vi "DPO 4034 Config Channel.vi"(4 "Bandwidth (0: FULL)":u16(ring) items=["FULL", "250 MHz", "150 MHz", "20 MHz"], 5 "Input Impedance (0: 1M ohm)":u16(ring) items=["1M", "75", "50"], 6 "Vertical Range (10.0 V)":dbl=10.0, 7 "Enable Channel (T: Enable)":bool=TRUE, 8 "error in (no error)":errorcluster, 9 "Vertical Coupling (1: DC)":u16(ring)=1 items=["AC", "DC", "Ground"], 10 "Channel (0: Channel 1)":u16(ring) items=["Channel 1", "Channel 2", "Channel 3", "Channel 4", "Math", "Reference 1", "Reference 2", "Reference 3", "Reference 4", "Bus 1", "Bus 2"], 11 "VISA resource name":refnum<visa-resource-name>) -> (0 "error out":errorcluster, 3 "VISA resource name out":refnum<visa-resource-name>)   [LabVIEW 2012]
panel:
  in  "Vertical Offset (0.0 V)":dbl
  in  "Probe Attenuation (1)":dbl=1.0
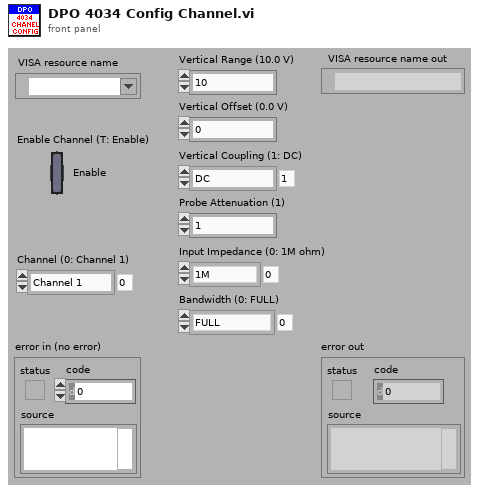
[diagram p1: front panel]
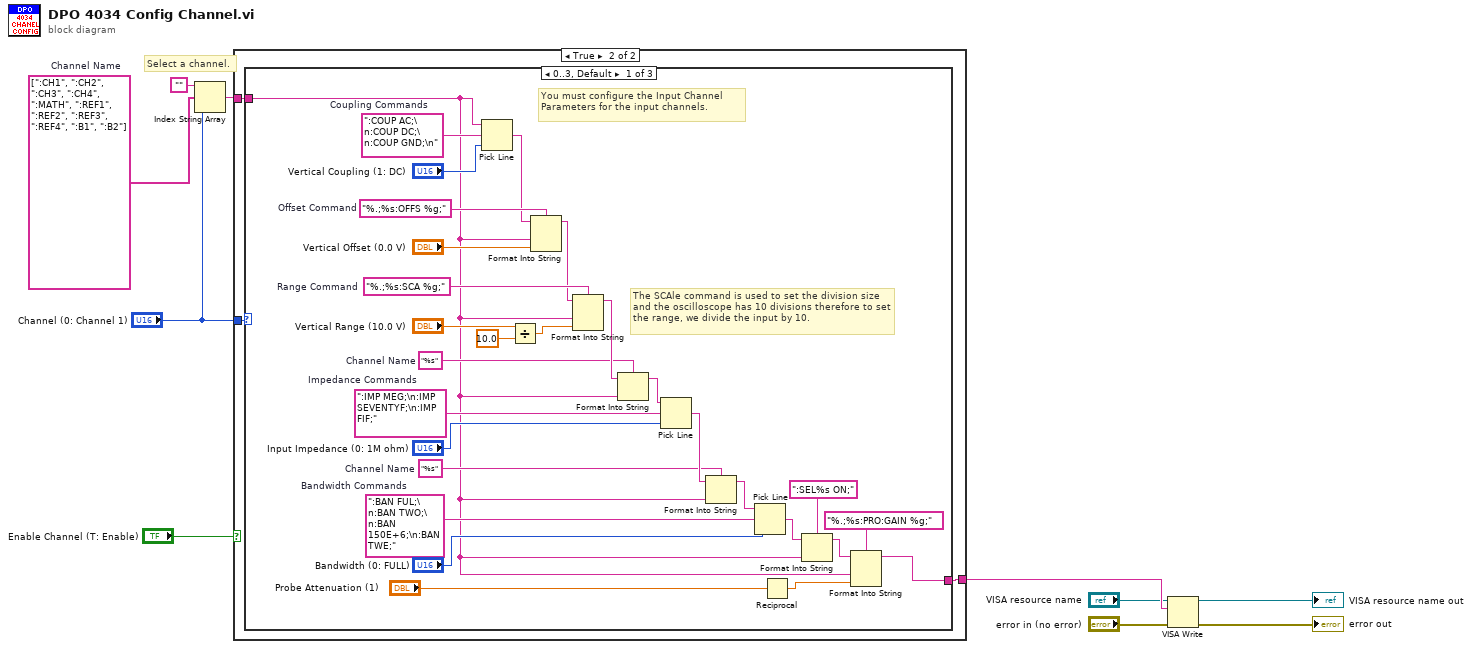
[diagram p0: block diagram]
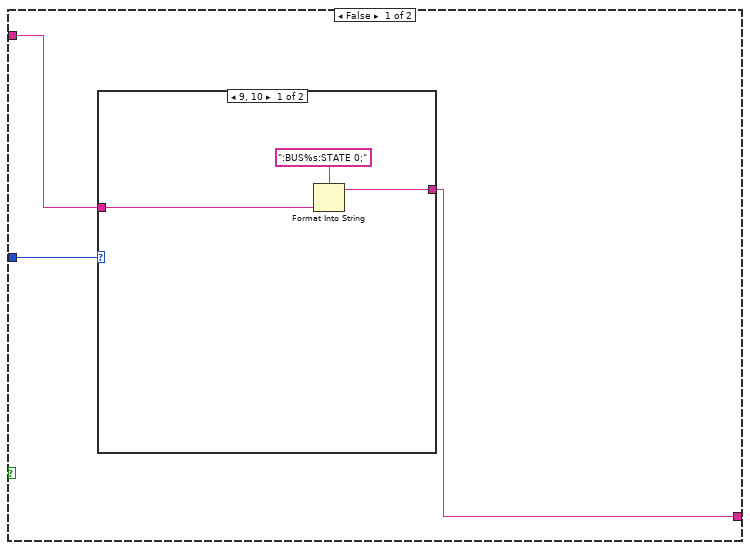
[diagram p2: hidden frame]
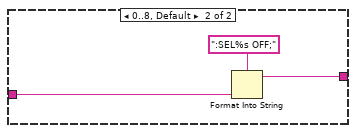
[diagram p3: hidden frame]
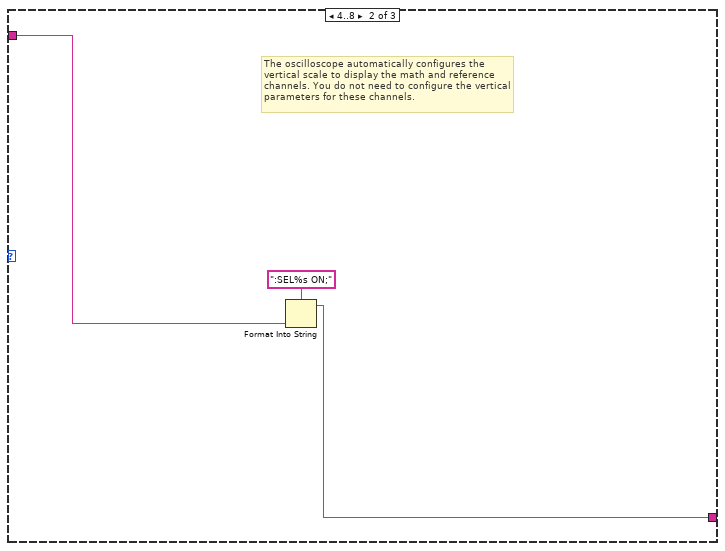
[diagram p4: hidden frame]
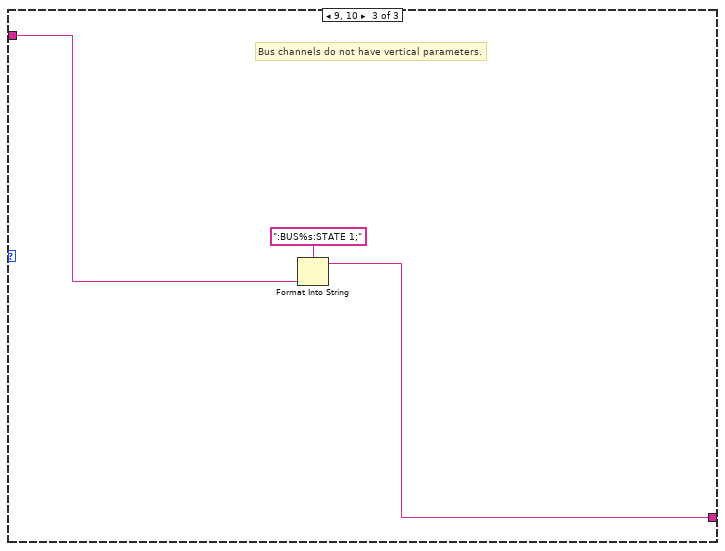
[diagram p5: hidden frame]
diagram:
  w7 = string[] [":CH1", ":CH2", ":CH3", ":CH4", ":MATH", ":REF1", ":REF2", ":REF3", ":REF4", ":B1", ":B2"]  # Channel Name
  # "Select a channel."
  n1 = Index String Array(1:"Channel (0: Channel 1)", 2:w7, 3:"") -> (0:w8:string)
  n2 = case shown="True" "Enable Channel (T: Enable)" {
    tunnel: w8 -> [w12 w21]
    tunnel: "Channel (0: Channel 1)" -> [w13 w22]
    tunnel: [w11 w20] -> w5
    frame False {
      n3 = case shown="9, 10" w13 {
        tunnel: w12 -> [w15 w18]
        tunnel: [w14 w17] -> w11
        frame 9, 10 {
          n4 = Format Into String(format string=":BUS%s:STATE 0;", w15) -> (resulting string=w14:string)  [unwired: 2 in, 1 out]
        }
        frame 0..8, Default {
          n5 = Format Into String(format string=":SEL%s OFF;", w18) -> (resulting string=w17:string)  [unwired: 2 in, 1 out]
        }
      }
    }
    frame True {
      n6 = case shown="0..3, Default" w22 {
        tunnel: w21 -> [w23 w51 w54]
        tunnel: [w26 w52 w55] -> w20
        frame 0..3, Default {
          w35 = ":BAN FUL;\n:BAN TWO;\n:BAN 150E+6;\n:BAN TWE;"  # Bandwidth Commands
          w37 = "%s"  # Channel Name
          w38 = "%s"  # Channel Name
          w40 = ":IMP MEG;\n:IMP SEVENTYF;\n:IMP FIF;"  # Impedance Commands
          w46 = "%.;%s:SCA %g;"  # Range Command
          w48 = "%.;%s:OFFS %g;"  # Offset Command
          w50 = ":COUP AC;\n:COUP DC;\n:COUP GND;\n"  # Coupling Commands
          # "The SCAle command is used to set the division size\nand the oscilloscope has 10 divisions therefore to set\nthe range, we divide the input by 10."
          # "You must configure the Input Channel\nParameters for the input channels."
          n7 = Pick Line(string ("")=w23, multi-line string=w50, line index="Vertical Coupling (1: DC)") -> (output string=w45:string)
          n8 = Divide(x="Vertical Range (10.0 V)", y=10.0) -> (x/y=w29:dbl)
          n9 = Format Into String(format string=w48, initial string=w45, w23, "Vertical Offset (0.0 V)") -> (resulting string=w44:string)  [unwired: 1 in, 1 out]
          n10 = Format Into String(format string=w46, initial string=w44, w23, w29) -> (resulting string=w42:string)  [unwired: 1 in, 1 out]
          n11 = Format Into String(format string=w38, initial string=w42, w23) -> (resulting string=w41:string)  [unwired: 1 in, 1 out]
          n12 = Pick Line(string ("")=w41, multi-line string=w40, line index="Input Impedance (0: 1M ohm)") -> (output string=w39:string)
          n13 = Format Into String(format string=w37, initial string=w39, w23) -> (resulting string=w36:string)  [unwired: 1 in, 1 out]
          n14 = Pick Line(string ("")=w36, multi-line string=w35, line index="Bandwidth (0: FULL)") -> (output string=w32:string)
          n15 = Reciprocal(x="Probe Attenuation (1)") -> (1/x=w25:dbl)
          n16 = Format Into String(format string=":SEL%s ON;", initial string=w32, w23) -> (resulting string=w28:string)  [unwired: 1 in, 1 out]
          n17 = Format Into String(format string="%.;%s:PRO:GAIN %g;", initial string=w28, w23, w25) -> (resulting string=w26:string)  [unwired: 1 in, 1 out]
        }
        frame 4..8 {
          # "The oscilloscope automatically configures the vertical scale to display the math and reference channels. You do not need to configure the vertical parameters for these channels."
          n18 = Format Into String(format string=":SEL%s ON;", w51) -> (resulting string=w52:string)  [unwired: 2 in, 1 out]
        }
        frame 9, 10 {
          # "Bus channels do not have vertical parameters."
          n19 = Format Into String(format string=":BUS%s:STATE 1;", w54) -> (resulting string=w55:string)  [unwired: 2 in, 1 out]
        }
      }
    }
  }
  n20 = VISA Write(VISA resource name="VISA resource name", write buffer=w5, error in (no error)="error in (no error)") -> (VISA resource name out=→"VISA resource name out":refnum<visa-resource-name>, error out=→"error out":errorcluster)  [unwired: 1 out]
